vi "create unique folder.vi"(10 "string":string, 11 "path 2":path) -> (3 "path":path)   [LabVIEW 2013]
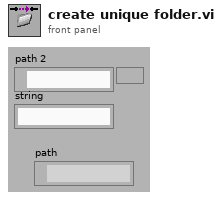
[diagram p1: front panel]
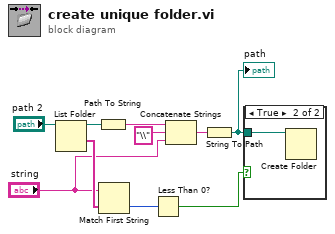
[diagram p0: block diagram]
diagram:
  n1 = List Folder(path="path 2") -> (path out=w7:path, folder names=w10:string[])  [unwired: 3 in, 2 out]
  n2 = Path To String(path=w7) -> (string=w6:string)
  n3 = Match First String(2:w10, 3:"string") -> (0:w9:i32)  [unwired: 1 out]
  n4 = Less Than 0?(x=w9) -> (x < 0?=w8:bool)
  n5 = Concatenate Strings(w6, "\\", "string") -> (w4:string)
  n6 = String To Path(string=w4) -> (path=w3:path)
  "path" <- w3
  n7 = case shown="True" w8 {
    tunnel: w3 -> [_ w11]
    frame False {
    }
    frame True {
      n8 = Create Folder(path (use dialog)=w11) -> ()  [unwired: 2 in, 3 out]
    }
  }
